vi "save_to_file.vi"() -> ()   [LabVIEW 2012]
uses:
  meas_date.vi
  <vilib>/Utility/file.llb/Write To Spreadsheet File (string).vi
panel:
  in  "Test ID":i32
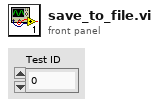
[diagram p1: front panel]
types:
  T1 = cluster{"VCT measurment's date":cluster{"No.":u64, "Voltage":dbl, "Current":dbl, "time":dbl, "Temperature":dbl}[], "Data":timestamp}[]
  T2 = cluster{"VCT measurment's date":cluster{"No.":u64, "Voltage":dbl, "Current":dbl, "time":dbl, "Temperature":dbl}[], "Data":timestamp}
  T3 = cluster{"No.":u64, "Voltage":dbl, "Current":dbl, "time":dbl, "Temperature":dbl}[]
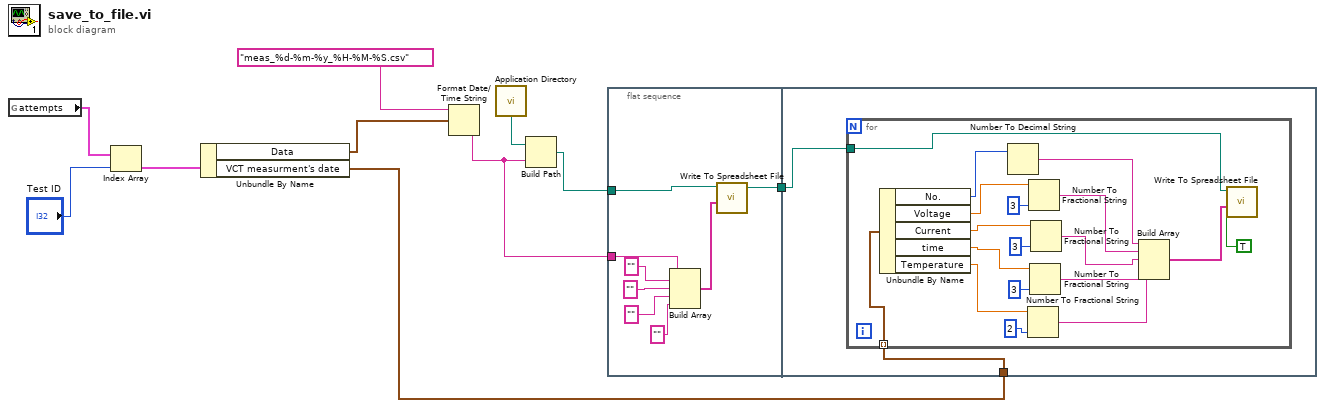
[diagram p0: block diagram]
diagram:
  n1 = global read "meas_date.vi" "attempts"() -> (w8:T1)
  n2 = Index Array(array=w8, index="Test ID") -> (element=w6:T2)
  n3 = Unbundle By Name(w6) -> ("Data"=w5:timestamp, "VCT measurment's date"=w2:T3)
  n4 = Format Date/Time String(time format string (%c)="meas_%d-%m-%y_%H-%M-%S.csv", seconds (now)=w5) -> (date/time string=w3:string)  [unwired: 1 in]
  n5 = call <vilib>:"Application Directory.vi"() -> ("Application Directory"=w9:path)
  n6 = Build Path(base path=w9, name or relative path=w3) -> (appended path=w4:path)
  n7 = flat-sequence {
    tunnel: w4 -> [w18]
    tunnel: w3 -> [w17]
    tunnel: [w11] -> w1
    tunnel: w2 -> [w20]
    tunnel: w1 -> [w19]
    frame #0 {
      n8 = Build Array(w17, "" ("element"), "" ("element"), "" ("element"), "" ("element")) -> (w12:string[])
      n9 = call-poly <vilib>:"Write To Spreadsheet File.vi"("1D data"=w12, "file path (dialog if empty)"=w18) -> ("new file path (Not A Path if cancelled)"=w11:path)  [unwired: 6 in]
    }
    frame #1 {
      n10 = for {
        tunnel: w20 -> [w24] mode=indexing
        tunnel: w19 -> [w22]
        n11 = Unbundle By Name(w24) -> ("No."=w38:u64, "Voltage"=w37:dbl, "Current"=w35:dbl, "time"=w32:dbl, "Temperature"=w31:dbl)
        n12 = Number To Decimal String(number=w38) -> (decimal integer string=w27:string)  [unwired: 1 in]
        n13 = Number To Fractional String(number=w31, precision (6)=i16 2) -> (F-format string=w29:string)  [unwired: 2 in]
        n14 = Number To Fractional String(number=w37, precision (6)=i16 3) -> (F-format string=w26:string)  [unwired: 2 in]
        n15 = Number To Fractional String(number=w32, precision (6)=i16 3) -> (F-format string=w28:string)  [unwired: 2 in]
        n16 = Number To Fractional String(number=w35, precision (6)=i16 3) -> (F-format string=w25:string)  [unwired: 2 in]
        n17 = Build Array(w27, w26, w25, w28, w29) -> (w21:string[])
        n18 = call-poly <vilib>:"Write To Spreadsheet File.vi"("append to file? (new file:F)"=TRUE, "1D data"=w21, "file path (dialog if empty)"=w22) -> ()  [unwired: 5 in, 1 out]
      }
    }
  }
